vi "20211224_HW1.vi"() -> ()   [LabVIEW 2019]
uses:
  Info.ctl
  <vilib>/Utility/miscctls.llb/LVPositionTypeDef.ctl
  Status.ctl
  Motion_Info.ctl
  3b30bc62-370e-4e5e-b0ed-d0be7c56b8e0.vi
panel:
  in  "Middle Ball":bool
  out "Right Ball":bool
  out "Deg":dbl
  out "Left Ball":bool
  out "2D Picture":picture
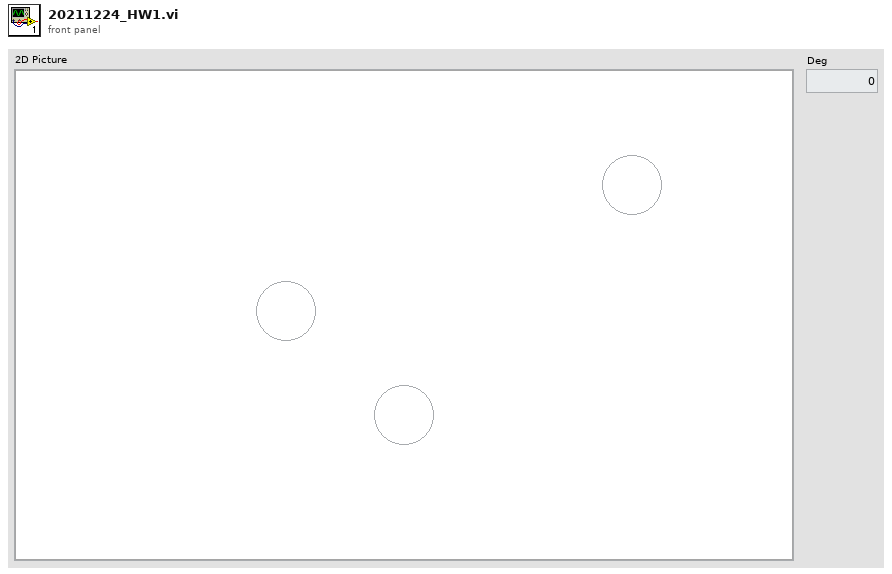
[diagram p1: front panel]
types:
  T1 = typedef "Motion_Info.ctl" = cluster{"Start Theta":dbl, "Period":dbl, "Start Time":u32}
  T2 = typedef "Status.ctl" = enum16{"Idle", "Motion"}
  T3 = cluster{"Width":u16, "Style":enum32{"Solid", "Dash", "Dot", "DashDot", "DashDotDot"}}
  T4 = typedef "LVPositionTypeDef.ctl" = cluster{"Left":i32, "Top":i32}
  T5 = typedef "Info.ctl" = cluster{"Start Drag":bool, "Position Offset":T4, "Theta Offset":dbl}
  T6 = typedef "LVBoundsTypeDef.ctl" = cluster{"Width":u32, "Height":u32}
  T7 = typedef "LVPoint32TypeDef.ctl" = cluster{"Horizontal":i32, "Vertical":i32}
  T8 = cluster{"Label.Bounds:Area Height":u32, "Label.Height":u32}
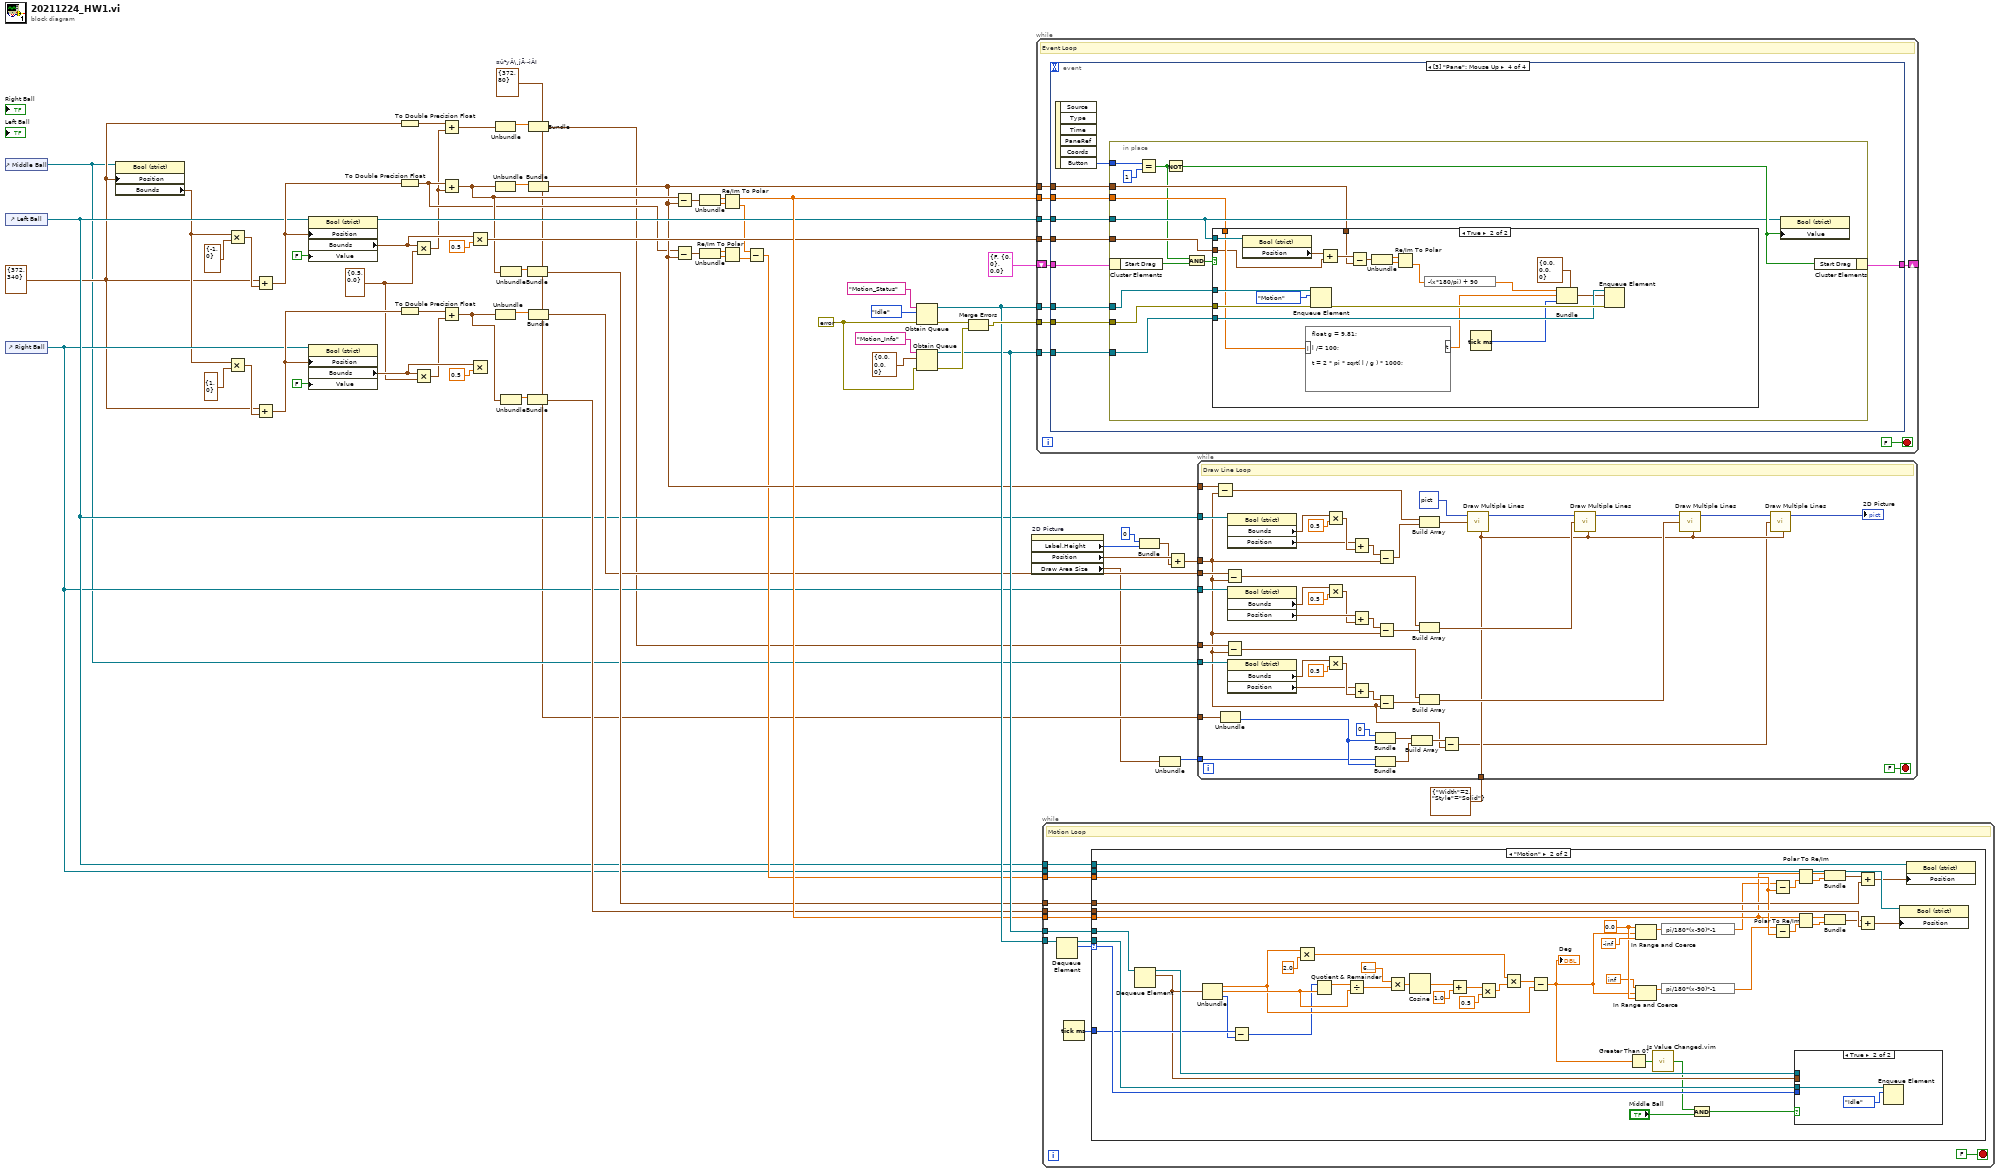
[diagram p0: block diagram]
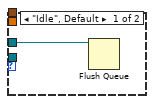
[diagram p2: hidden frame]
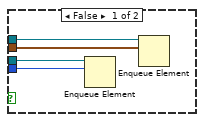
[diagram p3: hidden frame]
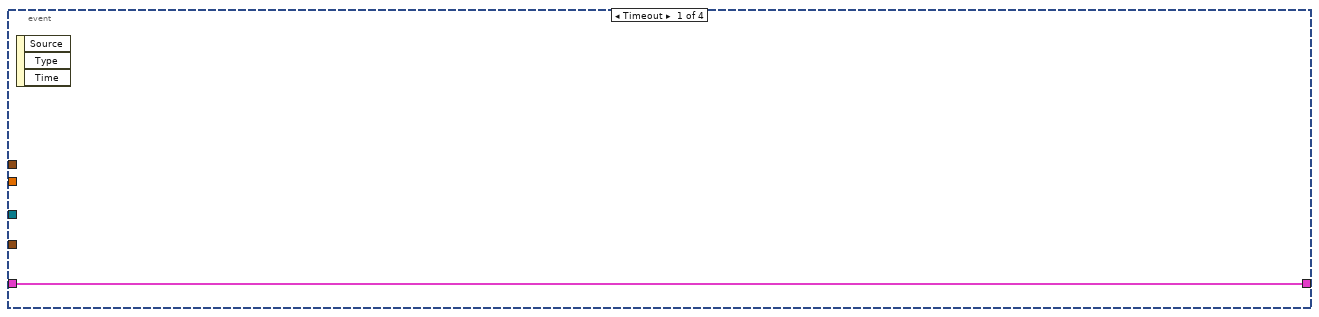
[diagram p4: hidden frame]
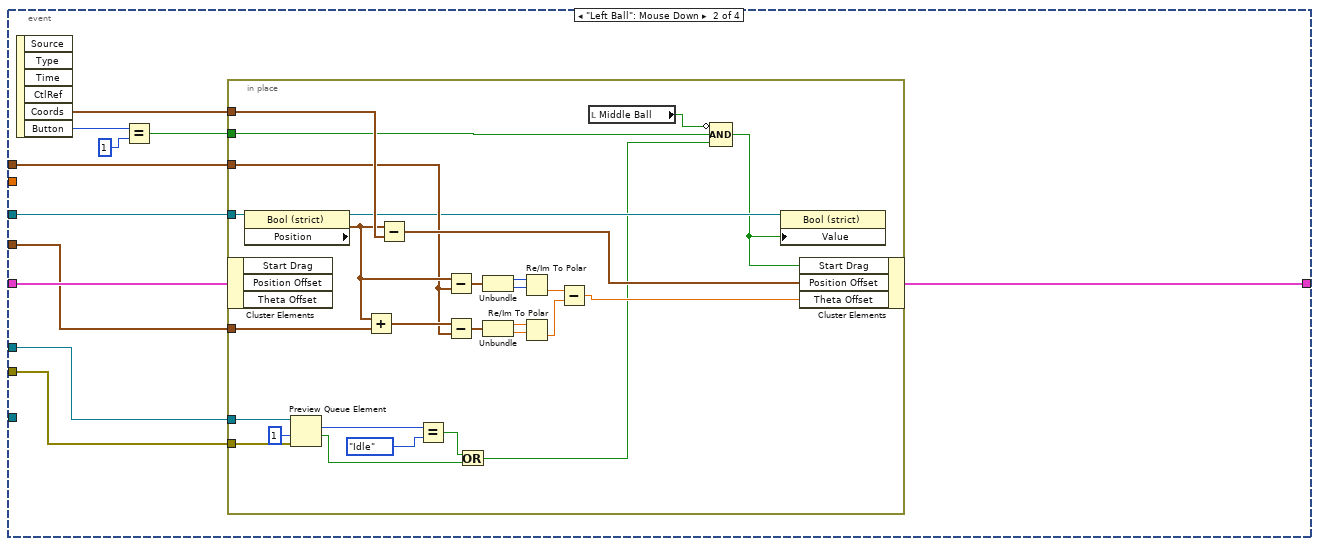
[diagram p5: hidden frame]
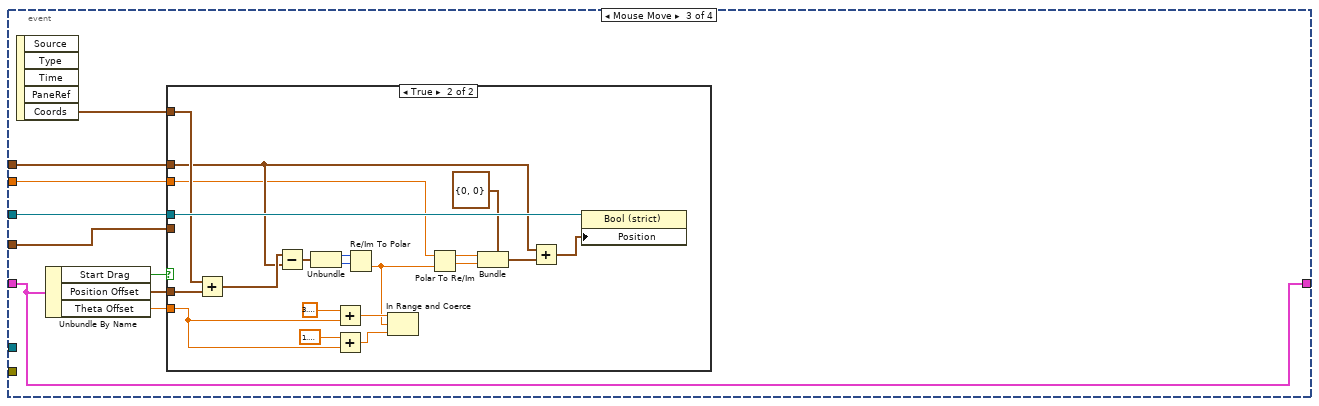
[diagram p6: hidden frame]
diagram:
  w52 = errorcluster {"status"=FALSE, "code"=0, "source"=""} ("error in (no error)")
  w17 = cluster{"Width":dbl, "Height":dbl} {"Width"=0.5, "Height"=0.0} ("y")
  w3 = T4 {"Left"=372, "Top"=80}  # ¤û¹yÂ\¸jÃ·­ìÂI
  w8 = T4 {"Left"=372, "Top"=340} ("Position")
  n1 = control-ref of="Middle Ball"() -> (w5:refnum<vi>)
  n2 = control-ref of="Left Ball"() -> (w14:refnum<vi>)
  n3 = control-ref of="Right Ball"() -> (w13:refnum<vi>)
  n4 = property class="Bool (strict)"(reference=w5, "Position"=w8) -> ("Bounds"=w12:T6)  [unwired: 1 in, 2 out]
  n5 = Multiply(x=w12, y=cluster{"Width":i32, "Height":i32} {"Width"=-1, "Height"=0}) -> (x*y=w30:T6)
  n6 = Multiply(x=w12, y=cluster{"Width":i32, "Height":i32} {"Width"=1, "Height"=0}) -> (x*y=w26:T6)
  n7 = Add(x=w8, y=w30) -> (x+y=w29:T6)
  n8 = Add(x=w8, y=w26) -> (x+y=w27:T6)
  n9 = property class="Bool (strict)"(reference=w14, "Position"=w29, "Value"=FALSE) -> (reference out=w44:refnum<vi>, "Bounds"=w32:T6)  [unwired: 1 in, 1 out]
  n10 = property class="Bool (strict)"(reference=w13, "Position"=w27, "Value"=FALSE) -> ("Bounds"=w24:T6)  [unwired: 1 in, 2 out]
  n11 = To Double Precision Float(number=w8) -> (double precision float=w11:cluster{"Left":dbl, "Top":dbl})
  n12 = To Double Precision Float(number=w29) -> (double precision float=w7:cluster{"Width":dbl, "Height":dbl})
  n13 = To Double Precision Float(number=w27) -> (double precision float=w28:cluster{"Width":dbl, "Height":dbl})
  n14 = Multiply(x=w32, y=w17) -> (x*y=w4:cluster{"Width":dbl, "Height":dbl})
  n15 = Multiply(x=w24, y=w17) -> (x*y=w19:cluster{"Width":dbl, "Height":dbl})
  n16 = Add(x=w11, y=w4) -> (x+y=w10:cluster{dbl, dbl})
  n17 = Add(x=w7, y=w4) -> (x+y=w42:cluster{"Width":dbl, "Height":dbl})
  n18 = Add(x=w28, y=w19) -> (x+y=w22:cluster{"Width":dbl, "Height":dbl})
  n19 = Multiply(x=w32, y=0.5 ("Width")) -> (x*y=w43:cluster{"Width":dbl, "Height":dbl})
  n20 = Multiply(x=w24, y=0.5 ("Width")) -> ()  [unwired: 1 out]
  n21 = Unbundle(w10) -> (w9:dbl)  [unwired: 1 out]
  n22 = Unbundle(w42) -> ("Width"=w67:dbl)  [unwired: 1 out]
  n23 = Unbundle(w22) -> ("Width"=w18:dbl)  [unwired: 1 out]
  n24 = Unbundle(w42) -> ("Width"=w41:dbl)  [unwired: 1 out]
  n25 = Unbundle(w22) -> ("Width"=w23:dbl)  [unwired: 1 out]
  n26 = Bundle(cluster=w3, "Left"=w41) -> (w40:T4)  [unwired: 1 in]
  n27 = Bundle(cluster=w3, "Left"=w23) -> (w15:T4)  [unwired: 1 in]
  n28 = Bundle(cluster=w3, "Left"=w9) -> (w6:T4)  [unwired: 1 in]
  n29 = Bundle(cluster=w3, "Left"=w67) -> (w37:T4)  [unwired: 1 in]
  n30 = Bundle(cluster=w3, "Left"=w18) -> (w16:T4)  [unwired: 1 in]
  n31 = Subtract(x=w42, y=w37) -> (x-y=w63:cluster{dbl, dbl})
  n32 = Subtract(x=w7, y=w37) -> (x-y=w39:cluster{dbl, dbl})
  n33 = Unbundle(w63) -> (w64:dbl, w65:dbl)
  n34 = Unbundle(w39) -> (w33:dbl, w38:dbl)
  n35 = Re/Im To Polar(2:w65, 3:w64) -> (0:w36:dbl, 1:w45:dbl)
  n36 = Re/Im To Polar(2:w38, 3:w33) -> (0:w35:dbl)  [unwired: 1 out]
  n37 = Subtract(x=w36, y=w35) -> (x-y=w34:dbl)
  n38 = Obtain Queue(name (unnamed)="Motion_Status", element data type=Status."Idle", error in (no error)=w52) -> (queue out=w47:refnum<queue>, error out=w50:errorcluster)  [unwired: 2 in, 1 out]
  n39 = Obtain Queue(name (unnamed)="Motion_Info", element data type=T1 {"Start Theta"=0.0, "Period"=0.0, "Start Time"=0}, error in (no error)=w52) -> (queue out=w46:refnum<queue>, error out=w49:errorcluster)  [unwired: 2 in, 1 out]
  n40 = Merge Errors(w50, w49) -> (w48:errorcluster)
  n41 = property on="2D Picture" class="Pict"() -> ("Label.Height"=w61:u32, "Position"=w59:T4, "Draw Area Size"=w2:T6)  [unwired: 2 in, 2 out]
  n42 = while {
    shift-right: [w75] -> _
    shift-left: T5 {"Start Drag"=FALSE, "Position Offset"={"Left"=0, "Top"=0}, "Theta Offset"=0.0} -> [w77]
    tunnel: w44 -> [w76]
    tunnel: w37 -> [w74]
    tunnel: w45 -> [w73]
    tunnel: w43 -> [w72]
    tunnel: w48 -> [w71]
    tunnel: w47 -> [w70]
    tunnel: w46 -> [w69]
    stop <- FALSE stop-if-true
    # "Event Loop"
    n43 = event shown="[3] \"Pane\": Mouse Up" {
      selector: _ -> [_ _ _ _]
      dyn-events: _ -> [_ _ _ _]
      timeout: _ -> [_ _ _ _]
      tunnel: w77 -> [w79 w90 w123 w156]
      tunnel: w76 -> [_ w88 w127 w154]
      tunnel: [w79 w89 w123 w155] -> w75
      tunnel: w74 -> [_ w86 w122 w150]
      tunnel: w73 -> [_ _ w121 w148]
      tunnel: w72 -> [_ w85 w120 w149]
      tunnel: w71 -> [_ w80 _ w153]
      tunnel: w70 -> [_ w81 _ w152]
      tunnel: w69 -> [_ _ _ w151]
      event Timeout {
        n44 = event-data() -> ()  [unwired: 1 in, 3 out]
      }
      event "Left Ball": Mouse Down {
        n45 = event-data() -> ("Coords"=w87:T7, "Button"=w83:u16)  [unwired: 1 in, 4 out]
        n46 = Equal?(x=w83, y=u16 1) -> (x = y?=w82:bool)
        n47 = in-place {
          in-place-border: w88 -> [w118]
          in-place-border: w87 -> [w117]
          in-place-border: w86 -> [w109]
          in-place-border: w85 -> [w112]
          in-place-border: w82 -> [w97]
          in-place-border: w81 -> [w101]
          in-place-border: w80 -> [w100]
          n48 = in-place-cluster #1(w90) -> ()  [unwired: 3 out]
          n49 = property class="Bool (strict)"(reference=w118) -> (reference out=w102:refnum<vi>, "Position"=w113:T4)  [unwired: 1 in, 1 out]
          n50 = Preview Queue Element(queue=w101, timeout in ms (-1)=1, error in (no error)=w100) -> (element=w99:T2, timed out?=w94:bool)  [unwired: 2 out]
          n51 = Add(x=w113, y=w112) -> (x+y=w110:cluster{dbl, dbl})
          n52 = Subtract(x=w113, y=w117) -> (x-y=w114:T4)
          n53 = Equal?(x=w99, y=Status."Idle") -> (x = y?=w93:bool)
          n54 = Subtract(x=w113, y=w109) -> (x-y=w111:T4)
          n55 = Subtract(x=w110, y=w109) -> (x-y=w108:cluster{dbl, dbl})
          n56 = Or(x=w93, y=w94) -> (x .or. y?=w92:bool)
          n57 = Unbundle(w111) -> ("Left"=w116:i32, "Top"=w115:i32)
          n58 = Unbundle(w108) -> (w107:dbl, w106:dbl)
          n59 = Re/Im To Polar(2:w115, 3:w116) -> (0:w105:dbl)  [unwired: 1 out]
          n60 = Re/Im To Polar(2:w106, 3:w107) -> (0:w104:dbl)  [unwired: 1 out]
          n61 = Subtract(x=w105, y=w104) -> (x-y=w103:dbl)
          n62 = local read "Middle Ball"() -> (w91:bool)
          n63 = Compound Arithmetic op=AND(invert w91, w97, w92) -> (w96:bool)
          n64 = property class="Bool (strict)"(reference=w102, "Value"=w96) -> ()  [unwired: 1 in, 2 out]
          n65 = in-place-cluster #1("Start Drag"=w96, "Position Offset"=w114, "Theta Offset"=w103) -> (w89:T5)
        }
      }
      event Mouse Move {
        n66 = event-data() -> ("Coords"=w126:T7)  [unwired: 1 in, 4 out]
        n67 = Unbundle By Name(w123) -> ("Start Drag"=w125:bool, "Position Offset"=w124:T4, "Theta Offset"=w119:dbl)
        n68 = case shown="True" w125 {
          tunnel: w127 -> [_ w147]
          tunnel: w126 -> [_ w143]
          tunnel: w124 -> [_ w141]
          tunnel: w122 -> [_ w136]
          tunnel: w121 -> [_ w135]
          tunnel: w120 -> [_ _]
          tunnel: w119 -> [_ w131]
          frame False {
          }
          frame True {
            n69 = Add(x=w143, y=w141) -> (x+y=w142:T7)
            n70 = Subtract(x=w142, y=w136) -> (x-y=w146:T7)
            n71 = Unbundle(w146) -> ("Horizontal"=w145:i32, "Vertical"=w144:i32)
            n72 = Add(x=3.141592653589793, y=w131) -> (x+y=w130:dbl)
            n73 = Add(x=1.5707963267948966, y=w131) -> (x+y=w129:dbl)
            n74 = Re/Im To Polar(2:w144, 3:w145) -> (0:w128:dbl)  [unwired: 1 out]
            n75 = In Range and Coerce(upper limit=w130, x=w128, lower limit=w129) -> ()  [unwired: 2 out]
            n76 = Polar To Re/Im(2:w128, 3:w135) -> (0:w139:dbl, 1:w140:dbl)
            n77 = Bundle(cluster=T4 {"Left"=0, "Top"=0} ("Position"), "Left"=w140, "Top"=w139) -> (w138:T4)
            n78 = Add(x=w136, y=w138) -> (x+y=w134:T4)
            n79 = property class="Bool (strict)"(reference=w147, "Position"=w134) -> ()  [unwired: 1 in, 2 out]
          }
        }
      }
      event Mouse Up {
        n80 = event-data() -> ("Button"=w157:u16)  [unwired: 1 in, 5 out]
        n81 = in-place {
          in-place-border: w157 -> [w170]
          in-place-border: w154 -> [w162]
          in-place-border: w153 -> [w166]
          in-place-border: w152 -> [w165]
          in-place-border: w151 -> [w163]
          in-place-border: w150 -> [w160]
          in-place-border: w149 -> [w161]
          in-place-border: w148 -> [w159]
          n82 = in-place-cluster #2(w156) -> ("Start Drag"=w168:bool)
          n83 = Equal?(x=w170, y=u16 1) -> (x = y?=w158:bool)
          n84 = Not(x=w158) -> (.not. x?=w167:bool)
          n85 = And(x=w158, y=w168) -> (x .and. y?=w164:bool)
          n86 = case shown="True" w164 {
            tunnel: w166 -> [_ w190]
            tunnel: w165 -> [_ w189]
            tunnel: w163 -> [_ w186]
            tunnel: w162 -> [_ w185]
            tunnel: w161 -> [_ w171]
            tunnel: w160 -> [_ w182]
            tunnel: w159 -> [_ w176]
            frame False {
            }
            frame True {
              n87 = property class="Bool (strict)"(reference=w185) -> ("Position"=w184:T4)  [unwired: 1 in, 2 out]
              n88 = formula code="float g = 9.81;\n\nl /= 100;\n\nt = 2 * pi * sqrt( l / g ) * 1000;"("l"=w176) -> ("t"=w175:dbl)
              n89 = Enqueue Element(queue=w189, element=Status."Motion", error in (no error)=w190) -> (error out=w187:errorcluster)  [unwired: 1 in, 2 out]
              n90 = Add(x=w184, y=w171) -> (x+y=w183:cluster{dbl, dbl})
              n91 = Subtract(x=w183, y=w182) -> (x-y=w181:cluster{dbl, dbl})
              n92 = Unbundle(w181) -> (w180:dbl, w179:dbl)
              n93 = Re/Im To Polar(2:w179, 3:w180) -> (0:w173:dbl)  [unwired: 1 out]
              n94 = expression code="-(x*180/pi) + 90"(w173) -> (w172:dbl)
              n95 = Tick Count (ms)() -> (millisecond timer value=w174:u32)
              n96 = Bundle(cluster=T1 {"Start Theta"=0.0, "Period"=0.0, "Start Time"=0}, "Start Theta"=w172, "Period"=w175, "Start Time"=w174) -> (w177:T1)
              n97 = Enqueue Element(queue=w186, element=w177, error in (no error)=w187) -> ()  [unwired: 1 in, 3 out]
            }
          }
          n98 = property class="Bool (strict)"(reference=w162, "Value"=w167) -> ()  [unwired: 1 in, 2 out]
          n99 = in-place-cluster #2("Start Drag"=w167) -> (w155:T5)
        }
      }
    }
  }
  n100 = while {
    tunnel: w47 -> [w202]
    tunnel: w46 -> [w199]
    tunnel: w45 -> [w196]
    tunnel: w40 -> [w195]
    tunnel: w14 -> [w194]
    tunnel: w34 -> [w193]
    tunnel: w13 -> [w192]
    tunnel: w15 -> [w191]
    stop <- FALSE stop-if-true
    # "Motion Loop"
    n101 = Dequeue Element(queue=w202) -> (queue out=w198:refnum<queue>, element=w200:T2)  [unwired: 2 in, 2 out]
    n102 = Tick Count (ms)() -> (millisecond timer value=w197:u32)
    n103 = case shown="\"Motion\"" w200 {
      selector: w200 -> [_ w250]
      tunnel: w199 -> [w203 w253]
      tunnel: w198 -> [_ w252]
      tunnel: w197 -> [_ w249]
      tunnel: w196 -> [_ w209]
      tunnel: w195 -> [_ w214]
      tunnel: w194 -> [_ w220]
      tunnel: w193 -> [_ w215]
      tunnel: w192 -> [_ w231]
      tunnel: w191 -> [_ w230]
      frame "Idle", Default {
        n104 = Flush Queue(queue=w203) -> ()  [unwired: 1 in, 3 out]
      }
      frame "Motion" {
        w211 = 0.0 ("upper limit")
        n105 = Dequeue Element(queue=w253) -> (queue out=w251:refnum<queue>, element=w248:T1)  [unwired: 2 in, 2 out]
        n106 = Unbundle(w248) -> ("Start Theta"=w240:dbl, "Period"=w246:dbl, "Start Time"=w247:u32)
        n107 = Subtract(x=w249, y=w247) -> (x-y=w238:u32)
        n108 = Multiply(x=w240, y=2.0) -> (x*y=w237:dbl)
        n109 = Quotient & Remainder(x=w238, y=w246) -> (x-y*floor(x/y)=w239:dbl)  [unwired: 1 out]
        n110 = Divide(x=w239, y=w246) -> (x/y=w244:dbl)
        n111 = Multiply(x=6.283185307179586, y=w244) -> (x*y=w243:dbl)
        n112 = Cosine(x=w243) -> (cos(x)=w236:dbl)
        n113 = Add(x=w236, y=1.0) -> (x+y=w234:dbl)
        n114 = Multiply(x=w234, y=0.5) -> (x*y=w232:dbl)
        n115 = Multiply(x=w237, y=w232) -> (x*y=w241:dbl)
        n116 = Subtract(x=w241, y=w240) -> (x-y=w208:dbl)
        "Deg" <- w208
        n117 = Greater Than 0?(x=w208) -> (x > 0?=w229:bool)
        n118 = In Range and Coerce(upper limit=w211, x=w208, lower limit=-inf) -> (coerced(x)=w207:dbl)  [unwired: 1 out]
        n119 = In Range and Coerce(upper limit=inf, x=w208, lower limit=w211) -> (coerced(x)=w206:dbl)  [unwired: 1 out]
        n120 = call "Is Value Changed.vim"("value"=w229) -> ("changed or first call?"=w228:bool)
        n121 = expression code="pi/180*(x-90)*-1"(w207) -> (w205:dbl)
        n122 = expression code="pi/180*(x-90)*-1"(w206) -> (w204:dbl)
        n123 = And(x=w228, y="Middle Ball") -> (x .and. y?=w226:bool)
        n124 = Subtract(x=w205, y=w215) -> (x-y=w219:dbl)
        n125 = Subtract(x=w204, y=w215) -> (x-y=w221:dbl)
        n126 = case shown="True" w226 {
          tunnel: w252 -> [w257 w259]
          tunnel: w251 -> [w256 _]
          tunnel: w250 -> [w255 _]
          tunnel: w248 -> [w254 _]
          frame False {
            n127 = Enqueue Element(queue=w257, element=w255) -> ()  [unwired: 2 in, 3 out]
            n128 = Enqueue Element(queue=w256, element=w254) -> ()  [unwired: 2 in, 3 out]
          }
          frame True {
            n129 = Enqueue Element(queue=w259, element=Status."Idle") -> ()  [unwired: 2 in, 3 out]
          }
        }
        n130 = Polar To Re/Im(2:w219, 3:w209) -> (0:w217:dbl, 1:w216:dbl)
        n131 = Polar To Re/Im(2:w221, 3:w209) -> (0:w224:dbl, 1:w225:dbl)
        n132 = Bundle(w216, w217) -> (w218:cluster{dbl, dbl})  [unwired: 1 in]
        n133 = Bundle(w225, w224) -> (w223:cluster{dbl, dbl})  [unwired: 1 in]
        n134 = Add(x=w218, y=w214) -> (x+y=w213:cluster{dbl, dbl})
        n135 = Add(x=w223, y=w230) -> (x+y=w222:cluster{dbl, dbl})
        n136 = property class="Bool (strict)"(reference=w231, "Position"=w222) -> ()  [unwired: 1 in, 2 out]
        n137 = property class="Bool (strict)"(reference=w220, "Position"=w213) -> ()  [unwired: 1 in, 2 out]
      }
    }
  }
  n138 = Bundle("Label.Bounds:Area Height"=u32 0, "Label.Height"=w61) -> (w58:T8)  [unwired: 1 in]
  n139 = Unbundle(w2) -> ("Width"=w1:u32)  [unwired: 1 out]
  n140 = Add(x=w59, y=w58) -> (x+y=w57:cluster{u32, u32})
  n141 = while {
    tunnel: w37 -> [w301]
    tunnel: w57 -> [w261]
    tunnel: T3 {"Width"=2, "Style"=enum."Solid"} ("pen") -> [w264]
    tunnel: w14 -> [w293]
    tunnel: w16 -> [w287]
    tunnel: w13 -> [w283]
    tunnel: w6 -> [w275]
    tunnel: w5 -> [w272]
    tunnel: w3 -> [w271]
    tunnel: w1 -> [w266]
    stop <- FALSE stop-if-true
    # "Draw Line Loop"
    n142 = Subtract(x=w301, y=w261) -> (x-y=w300:cluster{u32, u32})
    n143 = Unbundle(w271) -> ("Top"=w268:i32)  [unwired: 1 out]
    n144 = Subtract(x=w287, y=w261) -> (x-y=w285:cluster{u32, u32})
    n145 = Subtract(x=w275, y=w261) -> (x-y=w282:cluster{u32, u32})
    n146 = property on="Property Node" class="Bool (strict)"(reference=w293) -> ("Bounds"=w297:T6, "Position"=w296:T4)  [unwired: 1 in, 2 out]
    n147 = property on="Property Node" class="Bool (strict)"(reference=w283) -> ("Bounds"=w290:T6, "Position"=w291:T4)  [unwired: 1 in, 2 out]
    n148 = property on="Property Node" class="Bool (strict)"(reference=w272) -> ("Bounds"=w278:T6, "Position"=w277:T4)  [unwired: 1 in, 2 out]
    n149 = Multiply(x=w297, y=0.5 ("Width")) -> (x*y=w303:cluster{"Width":dbl, "Height":dbl})
    n150 = Multiply(x=w290, y=0.5 ("Width")) -> (x*y=w288:cluster{"Width":dbl, "Height":dbl})
    n151 = Multiply(x=w278, y=0.5 ("Width")) -> (x*y=w280:cluster{"Width":dbl, "Height":dbl})
    n152 = Add(x=w296, y=w303) -> (x+y=w295:cluster{dbl, dbl})
    n153 = Add(x=w291, y=w288) -> (x+y=w292:cluster{dbl, dbl})
    n154 = Add(x=w277, y=w280) -> (x+y=w276:cluster{dbl, dbl})
    n155 = Bundle("Left"=0, "Top"=w268) -> (w269:cluster{"Left":i32, "Top":i32})  [unwired: 1 in]
    n156 = Bundle("Width"=w266, "Top"=w268) -> (w267:cluster{"Width":u32, "Top":i32})  [unwired: 1 in]
    n157 = Subtract(x=w295, y=w261) -> (x-y=w298:cluster{dbl, dbl})
    n158 = Subtract(x=w292, y=w261) -> (x-y=w286:cluster{dbl, dbl})
    n159 = Subtract(x=w276, y=w261) -> (x-y=w281:cluster{dbl, dbl})
    n160 = Build Array(w269, w267) -> (w262:cluster{"Width":u32, "Top":i32}[])
    n161 = Build Array(w300, w298) -> (w302:cluster{dbl, dbl}[])
    n162 = Build Array(w285, w286) -> (w284:cluster{dbl, dbl}[])
    n163 = Build Array(w282, w281) -> (w273:cluster{dbl, dbl}[])
    n164 = Subtract(x=w262, y=w261) -> (x-y=w260:cluster{u32, u32}[])
    n165 = call <vilib>:"Draw Multiple Lines.vi"("picture"=picture data[5B], "line endpoints"=w302, "pen"=w264) -> ("new picture"=w294:picture)  [unwired: 6 in]
    n166 = call <vilib>:"Draw Multiple Lines.vi"("picture"=w294, "line endpoints"=w284, "pen"=w264) -> ("new picture"=w274:picture)  [unwired: 6 in]
    n167 = call <vilib>:"Draw Multiple Lines.vi"("picture"=w274, "line endpoints"=w273, "pen"=w264) -> ("new picture"=w265:picture)  [unwired: 6 in]
    n168 = call <vilib>:"Draw Multiple Lines.vi"("picture"=w265, "line endpoints"=w260, "pen"=w264) -> ("new picture"=→"2D Picture":picture)  [unwired: 6 in]
  }
